vi "Return ID to Pool.vi"(8 "error in (no error)":errorcluster, 9 "timeout in ms (0)":i32 format="%d ms", 10 "id":i32, 11 "ID Pool in":refnum<class "Pool ID.lvclass">) -> (0 "error out":errorcluster, 1 "timed out?":bool, 3 "ID Pool out":refnum<class "Pool ID.lvclass">)   [LabVIEW 2017, in "Data Sharing Framework Engine.lvlib" / "Pool ID.lvclass"]
uses:
  Pool ID.lvclass
  C:/github/data-sharing-framework/old/dsf core/Source/Engine/Classes/Thread Pool/Pool.lvclass
  Pool/Pool.lvclass/Pool.ctl
  Debug/Debug Flags FIFO/Debug Flags FIFO.lvclass/Debug Flags FIFO.ctl
  Pool/Get FIFO.vi
  Pool/Get Debug Flags.vi
  Debug/Debug Flags FIFO/Get Infinite Timeouts.vi
  Pool/Pool.lvclass
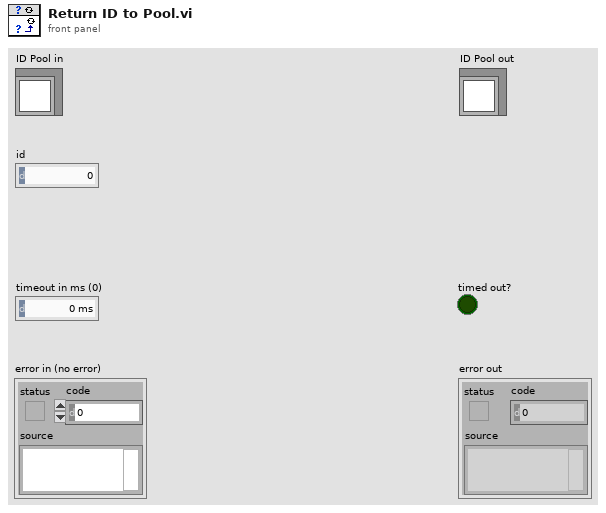
[diagram p1: front panel]
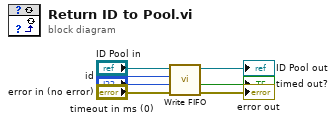
[diagram p0: block diagram]
diagram:
  n1 = call "Write FIFO.vi"("error in (no error)"="error in (no error)", "timeout in ms (0)"="timeout in ms (0)", "element"="id", "Pool in"="ID Pool in") -> ("error out"=→"error out":errorcluster, "timed out?"=→"timed out?":bool, "Pool out"=→"ID Pool out":refnum<class "Pool ID.lvclass">)  [unwired: 5 in]
